vi "Set Integration Time.vi"(8 "error in (no error)":errorcluster, 10 "Integration Time":dbl, 11 "Agilent 3458A in":refnum<class "Agilent 3458A.lvclass">) -> (0 "error out":errorcluster, 3 "Agilent 3458A out":refnum<class "Agilent 3458A.lvclass">)   [LabVIEW 2011, in "Agilent 3458A.lvclass"]
uses:
  Agilent 3458A.lvclass
  Measurement Integration.ctl
  <instrlib>/Agilent 3458/Agilent 3458.lvlib
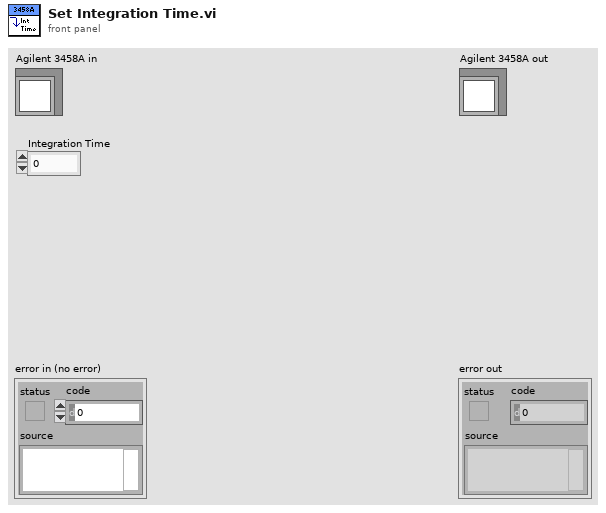
[diagram p1: front panel]
types:
  T1 = typedef "Agilent 3458A.lvclass/Measurement Integration.ctl" = cluster{"Power Line Cycles":dbl}
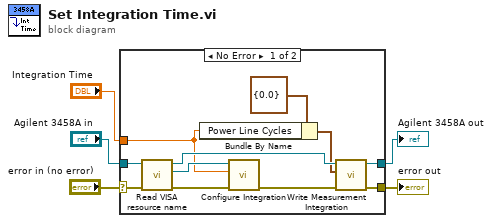
[diagram p0: block diagram]
diagram:
  n1 = case shown="No Error" "error in (no error)" {
    selector: "error in (no error)" -> [w14 w18]
    tunnel: [w11 w18] -> w4
    tunnel: [w10 w17] -> w2
    tunnel: "Agilent 3458A in" -> [w16 w17]
    tunnel: "Integration Time" -> [w7 _]
    frame No Error {
      n2 = call-dynamic "Read VISA resource name.vi"("error in (no error)"=w14, "Multimeter in"=w16) -> ("error out"=w13:errorcluster, "VISA resource name"=w15:refnum<visa-resource-name>, "Multimeter out"=w9:refnum<class "Agilent 3458A.lvclass">)  [unwired: 7 in]
      n3 = Bundle By Name(cluster=T1 {"Power Line Cycles"=0.0} ("Measurement Integration"), "Power Line Cycles"=w7) -> (w6:T1)
      n4 = call <instrlib>:"Configure Integration.vi"("error in (no error)"=w13, "Integration Time (0 PLCs)"=w7, "VISA resource name"=w15) -> ("error out"=w12:errorcluster)  [unwired: 7 in, 1 out]
      n5 = call-dynamic "Write Measurement Integration.vi"("error in (no error)"=w12, "Measurement Integration"=w6, "Agilent 3458A in"=w9) -> ("error out"=w11:errorcluster, "Agilent 3458A out"=w10:refnum<class "Agilent 3458A.lvclass">)  [unwired: 7 in]
    }
    frame Error {
    }
  }
  "error out" <- w4
  "Agilent 3458A out" <- w2
